vi "SR830_Source_Ramp_Algorithm.vi"(4 "Total Time (s)":dbl, 5 "Number of Steps":i32 step=1, 6 "Ref Level To":dbl, 7 "Ref Level From":dbl, 8 "error in (no error)":errorcluster, 9 "Waveform Chart Reference":refnum<vi>, 10 "Voltage Display\nReference":refnum<vi>[](array[refnum]), 11 "VISA resource name":refnum<visa-resource-name>) -> (0 "error out":errorcluster, 3 "VISA resource name out":refnum<visa-resource-name>)   [LabVIEW 2018]
uses:
  <instrlib>/Stanford Research 830/Stanford Research 830.lvlib
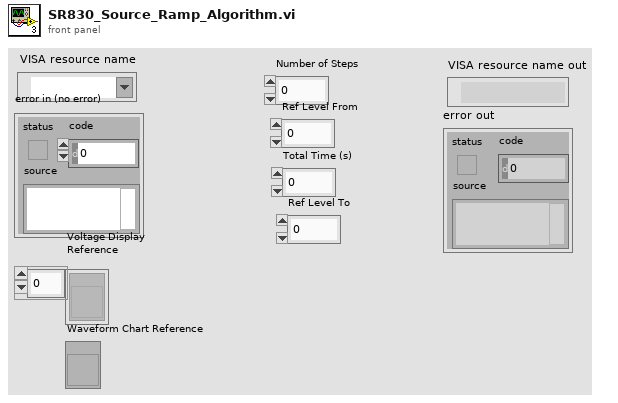
[diagram p1: front panel]
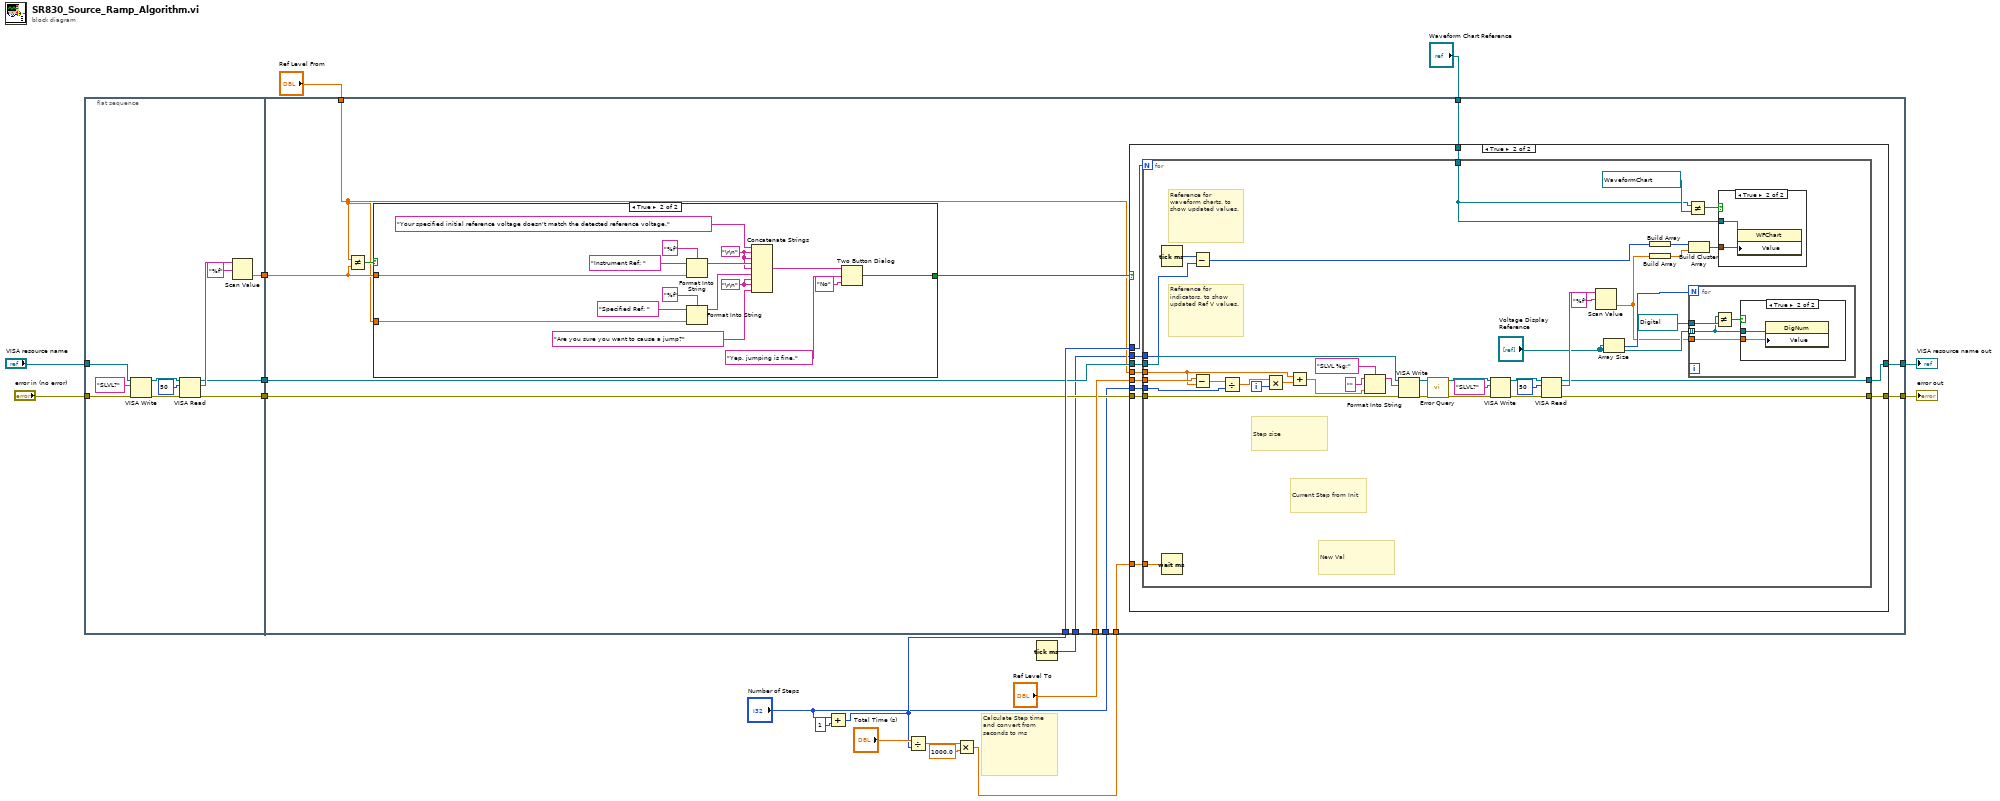
[diagram p0: block diagram]
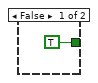
[diagram p5: hidden frame]
diagram:
  # "Calculate Step time and convert from seconds to ms"
  n1 = flat-sequence {
    tunnel: "VISA resource name" -> [w24]
    tunnel: "error in (no error)" -> [w23]
    tunnel: [w21] -> w16
    tunnel: [w20] -> w7
    tunnel: [w19] -> w6
    tunnel: w16 -> [w40]
    tunnel: "Ref Level From" -> [w33]
    tunnel: w11 -> [w41]
    tunnel: "Ref Level To" -> [w39]
    tunnel: w9 -> [w38]
    tunnel: w7 -> [w37]
    tunnel: w6 -> [w36]
    tunnel: [w35] -> w5
    tunnel: [w34] -> w4
    tunnel: "Number of Steps" -> [w32]
    tunnel: w2 -> [w31]
    tunnel: "Waveform Chart Reference" -> [w30]
    frame #0 {
      n2 = VISA Write(VISA resource name=w24, write buffer="SLVL?", error in (no error)=w23) -> (VISA resource name out=w22:refnum<visa-resource-name>, error out=w29:errorcluster)  [unwired: 1 out]
      n3 = VISA Read(VISA resource name=w22, byte count=u32 50, error in (no error)=w29) -> (VISA resource name out=w20:refnum<visa-resource-name>, read buffer=w25:string, error out=w19:errorcluster)  [unwired: 1 out]
      n4 = Scan Value(string=w25, format string="%f") -> (value=w21:dbl)  [unwired: 1 in, 1 out]
    }
    frame #1 {
      n5 = Not Equal?(x=w33, y=w40) -> (x != y?=w43:bool)
      n6 = case shown="True" w43 {
        tunnel: w33 -> [_ w107]
        tunnel: w40 -> [_ w110]
        tunnel: [TRUE ("T button?") w111] -> w42
        frame False {
        }
        frame True {
          w108 = "\r\n"
          w105 = "\r\n"
          n7 = Format Into String(format string="%f", initial string="Instrument Ref: ", w110) -> (resulting string=w113:string)  [unwired: 1 in, 1 out]
          n8 = Format Into String(format string="%f", initial string="Specified Ref: ", w107) -> (resulting string=w112:string)  [unwired: 1 in, 1 out]
          n9 = Concatenate Strings("Your specified initial reference voltage doesn't match the detected reference voltage." ("message"), w105, w105, w113, w105, w112, w108, w108, "Are you sure you want to cause a jump?" ("string")) -> (w118:string)
          n10 = Two Button Dialog(message=w118, 1:"No" ("F button name (\"Cancel\")"), 2:"Yep, jumping is fine." ("T button name (\"OK\")")) -> (T button?=w111:bool)
        }
      }
      n11 = case shown="True" w42 {
        tunnel: w41 -> [_ w56]
        tunnel: w33 -> [_ w55]
        tunnel: w39 -> [_ w54]
        tunnel: w38 -> [_ w53]
        tunnel: w37 -> [w45 w52]
        tunnel: w36 -> [w44 w51]
        tunnel: [w45 w50] -> w35
        tunnel: [w44 w49] -> w34
        tunnel: w32 -> [_ w48]
        tunnel: w31 -> [_ w47]
        tunnel: w30 -> [_ w46]
        frame False {
        }
        frame True {
          n12 = for {
            N: w56 -> [_]
            tunnel: w55 -> [w90]
            tunnel: w54 -> [w94]
            tunnel: w53 -> [w89]
            tunnel: w52 -> [w83]
            tunnel: w51 -> [w82]
            tunnel: [w72] -> w50
            tunnel: [w71] -> w49
            tunnel: w48 -> [w70]
            tunnel: w47 -> [w63]
            tunnel: w46 -> [w58]
            i -> [w95]
            # "Reference for waveform charts, to show updated values."
            # "Reference for indicators, to show updated Ref V values."
            # "New Val"
            # "Current Step from Init"
            # "Step size"
            n13 = Tick Count (ms)() -> (millisecond timer value=w64:u32)
            n14 = Wait (ms)(milliseconds to wait=w89) -> ()  [unwired: 1 out]
            n15 = Subtract(x=w64, y=w63) -> (x-y=w62:u32)
            n16 = Subtract(x=w94, y=w90) -> (x-y=w93:dbl)
            n17 = Divide(x=w93, y=w70) -> (x/y=w91:dbl)
            n18 = Multiply(x=w91, y=w95) -> (x*y=w92:dbl)
            n19 = Add(x=w90, y=w92) -> (x+y=w81:dbl)
            n20 = Format Into String(format string="SLVL %g;" ("write buffer"), initial string="", w81) -> (resulting string=w84:string)  [unwired: 1 in, 1 out]
            n21 = VISA Write(VISA resource name=w83, write buffer=w84, error in (no error)=w82) -> (VISA resource name out=w88:refnum<visa-resource-name>, error out=w87:errorcluster)  [unwired: 1 out]
            n22 = call <instrlib>:"Error Query.vi"("error in (no error)"=w87, "VISA resource name"=w88) -> ("error out"=w74:errorcluster, "VISA resource name out"=w73:refnum<visa-resource-name>)  [unwired: 7 in, 1 out]
            n23 = VISA Write(VISA resource name=w73, write buffer="SLVL?", error in (no error)=w74) -> (VISA resource name out=w75:refnum<visa-resource-name>, error out=w80:errorcluster)  [unwired: 1 out]
            n24 = VISA Read(VISA resource name=w75, byte count=u32 50, error in (no error)=w80) -> (VISA resource name out=w72:refnum<visa-resource-name>, read buffer=w76:string, error out=w71:errorcluster)  [unwired: 1 out]
            n25 = Scan Value(string=w76, format string="%f") -> (value=w60:dbl)  [unwired: 1 in, 1 out]
            n26 = Array Size(array="Voltage Display\nReference") -> (size(s)=w69:i32)
            n27 = Build Array(w62) -> (w61:u32[])
            n28 = Build Array(w60) -> (w59:dbl[])
            n29 = Not Equal?(x=w58, y=refnum<vi> refnum) -> (x != y?=w66:bool)
            n30 = Build Cluster Array(w61, w59) -> (w57:cluster{u32, dbl}[])
            n31 = for {
              N: w69 -> [_]
              tunnel: w60 -> [w101]
              tunnel: refnum<vi> refnum ("y") -> [w100]
              tunnel: "Voltage Display\nReference" -> [w98] mode=indexing
              n32 = Not Equal?(x=w98, y=w100) -> (x != y?=w99:bool)
              n33 = case shown="True" w99 {
                tunnel: w101 -> [_ w103]
                tunnel: w98 -> [_ w102]
                frame False {
                }
                frame True {
                  n34 = property class="DigNum"(reference=w102, "Value"=w103) -> ()  [unwired: 1 in, 2 out]
                }
              }
            }
            n35 = case shown="True" w66 {
              tunnel: w58 -> [_ w97]
              tunnel: w57 -> [_ w96]
              frame False {
              }
              frame True {
                n36 = property class="WFChart"(reference=w97, "Value"=w96) -> ()  [unwired: 1 in, 2 out]
              }
            }
          }
        }
      }
    }
  }
  n37 = Add(x="Number of Steps", y=1) -> (x+y=w11:i32)
  n38 = Divide(x="Total Time (s)", y=w11) -> (x/y=w8:dbl)
  n39 = Multiply(x=w8, y=1000.0) -> (x*y=w9:dbl)
  n40 = Tick Count (ms)() -> (millisecond timer value=w2:u32)
  "error out" <- w4
  "VISA resource name out" <- w5
